vi "Read Control Description.vi"(8 "error in (no error)":errorcluster, 9 "variant":variant) -> (0 "error out":errorcluster, 3 "VI Description":string)   [LabVIEW 2019, in "JSON-Schema.lvlib"]
uses:
  JSON-Schema.lvlib
  <vilib>/Utility/Data Type/NI_Data Type.lvlib
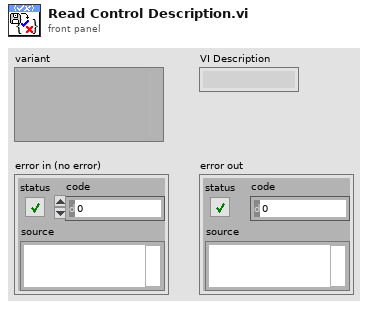
[diagram p1: front panel]
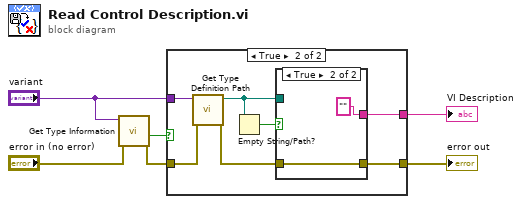
[diagram p0: block diagram]
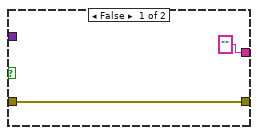
[diagram p2: hidden frame]
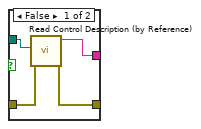
[diagram p3: hidden frame]
diagram:
  n1 = call <vilib>:"Get Type Information.vi"("error in (no error)"="error in (no error)", "variant"="variant") -> ("error out"=w2:errorcluster, "type definition"=w1:bool)  [unwired: 5 in, 3 out]
  n2 = case shown="True" w1 {
    tunnel: [w7 w11] -> w6
    tunnel: ["" ("VI Description") w15] -> w5
    tunnel: "variant" -> [_ w13]
    tunnel: w2 -> [w7 w12]
    frame False {
    }
    frame True {
      n3 = call <vilib>:"Get Type Definition Path.vi"("error in (no error)"=w12, "variant"=w13) -> ("error out"=w14:errorcluster, "type definition path"=w9:path)  [unwired: 8 in]
      n4 = Empty String/Path?(string/path=w9) -> (empty?=w10:bool)
      n5 = case shown="True" w10 {
        tunnel: [w17 "" ("VI Description")] -> w15
        tunnel: w14 -> [w19 w21]
        tunnel: w9 -> [w16 _]
        tunnel: [w18 w21] -> w11
        frame False {
          n6 = call "Read Control Description (by Reference).vi"("error in (no error)"=w19, "ctl path"=w16) -> ("error out"=w18:errorcluster, "VI Description"=w17:string)  [unwired: 7 in, 1 out]
        }
        frame True {
        }
      }
    }
  }
  "error out" <- w6
  "VI Description" <- w5
